vi "Reinit.vi"(6 "ACK":bool, 8 "error in":errorcluster) -> (0 "error out":errorcluster)   [LabVIEW 2015, in "Generic Module Library.lvlib" / "Template G_Module.lvlib"]
uses:
  Template G_Module.lvlib
  Private Controls/Module Message Cluster Components/Message Data Cluster.ctl
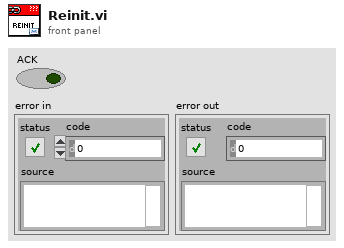
[diagram p1: front panel]
types:
  T1 = typedef "Generic Module Library.lvlib/Template G_Module.lvlib/Message Data Cluster.ctl" = cluster{"Module Action":string, "Message Data":variant}
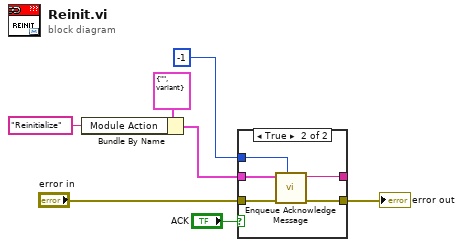
[diagram p0: block diagram]
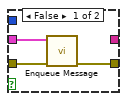
[diagram p2: hidden frame]
diagram:
  n1 = Bundle By Name(cluster=T1 {"Module Action"="", "Message Data"=variant} ("Message Data"), "Module Action"="Reinitialize") -> (w4:T1)
  n2 = case shown="True" "ACK" {
    tunnel: "error in" -> [w10 w15]
    tunnel: [w9 w14] -> w6
    tunnel: w4 -> [w8 w13]
    tunnel: -1 ("Ack Timeout") -> [_ w12]
    tunnel: [_ w11] -> _
    frame False {
      n3 = call "Enqueue Message.vi"("error in"=w10, "Message Data"=w8) -> ("error out"=w9:errorcluster)  [unwired: 9 in]
    }
    frame True {
      n4 = call "Enqueue Acknowledge Message.vi"("Ack Timeout"=w12, "error in"=w15, "Message Data"=w13) -> ("error out"=w14:errorcluster, "Response Data"=w11:string)  [unwired: 6 in, 1 out]
    }
  }
  "error out" <- w6
